vi "SetRenderDrawColor.vi"(4 "a":u8, 6 "b":u8, 8 "No Error":errorcluster, 9 "g":u8, 10 "r":u8, 11 "Renderer [SDL_Renderer *]":i64 format="%.0x") -> (0 "error out":errorcluster)   [LabVIEW 2026, in "SDL3.lvlib" / "Render.lvlib"]
doc: "<B>Summary</B>\nSet the color used for drawing operations."
uses:
  Render.lvlib
  <vilib>/Utility/error.llb/Error Cluster From Error Code.vi
  Error/Error.lvlib
  Lib/SDL3.dll
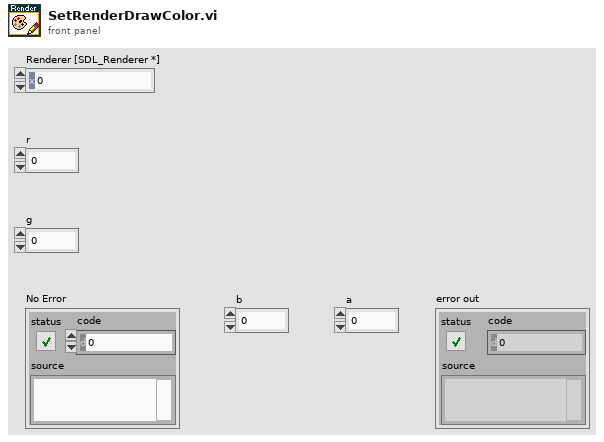
[diagram p1: front panel]
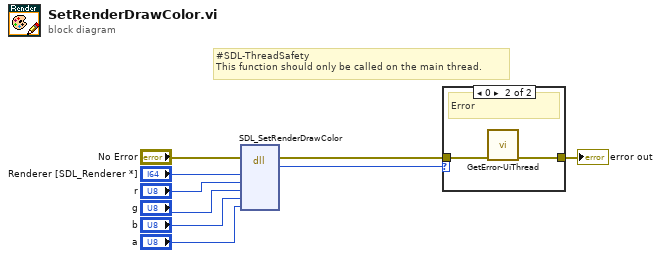
[diagram p0: block diagram]
diagram:
  # "#SDL-ThreadSafety\nThis function should only be called on the main thread."
  n1 = dll-call lib="C:/Users/saukko/Dev/LV-SDL3/Sources/SDL3/Lib/SDL3.*" fn="SDL_SetRenderDrawColor"(error in="No Error", "renderer"="Renderer [SDL_Renderer *]", "r"="r", "g"="g", "b"="b", "a"="a") -> (error out=w2:errorcluster, "return type"=w1:i32)  [unwired: 7 in, 1 out]
  n2 = case shown="0" w1 {
    tunnel: w2 -> [w10 w12]
    tunnel: [w10 w11] -> w8
    frame Default {
      # "Ok"
    }
    frame 0 {
      # "Error"
      n3 = call "GetError-UiThread.vi"("No Error"=w12) -> ("error out"=w11:errorcluster)  [unwired: 10 in]
    }
  }
  "error out" <- w8
